vi "Thermocouple DAQ Setup.vi"(0 "task in":refnum<k21>, 1 "sample mode":i32(ring)=10123 items=["Finite Samples"=10178, "Continuous Samples"=10123, "Hardware Timed Single Point"=12522], 3 "Thermocouple Type":i32(ring)=10073 items=["J"=10072, "K"=10073, "N"=10077, "R"=10082, "S"=10085, "T"=10086, "B"=10047, "E"=10055], 5 "physical channels":tag, 7 "Sample Rate":dbl=1000.0 format="%0.2f", 9 "minimum value":dbl format="%0.2f", 11 "error in":errorcluster, 12 "samples per channel":i32=1) -> (4 "task out":refnum<k21>, 15 "error out":errorcluster)   [LabVIEW 2016]
uses:
  <vilib>/DAQmx/create/channels.llb/DAQmx Create Channel (AI-Temperature-Thermocouple).vi
  <vilib>/DAQmx/configure/timing.llb/DAQmx Timing (Sample Clock).vi
panel:
  in  "maximum value":dbl=100.0 format="%0.2f"
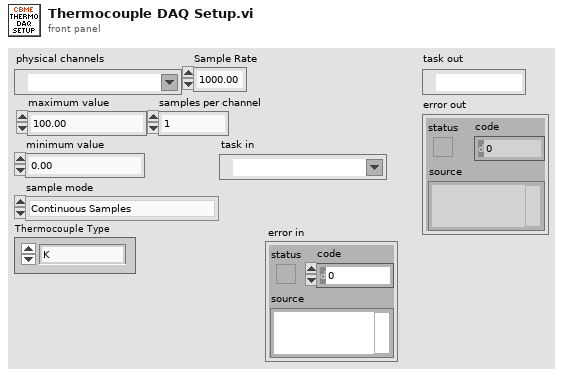
[diagram p1: front panel]
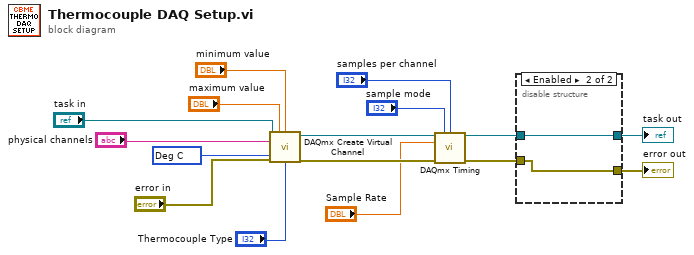
[diagram p0: block diagram]
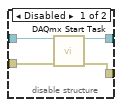
[diagram p2: hidden frame]
diagram:
  w13 = 10143 items=["Deg C"=10143, "Deg F"=10144, "Kelvins"=10325, "Deg R"=10145, "From Custom Scale"=10065] ("units")
  n1 = call-poly <vilib>:"DAQmx Create Virtual Channel.vi"("task in"="task in", "maximum value"="maximum value", "minimum value"="minimum value", "physical channels"="physical channels", "units"=w13, "error in"="error in", "thermocouple type"="Thermocouple Type") -> ("task out"=w12:refnum<k21>, "error out"=w11:errorcluster)  [unwired: 7 in]
  n2 = call-poly <vilib>:"DAQmx Timing.vi"("task/channels in"=w12, "sample mode"="sample mode", "samples per channel"="samples per channel", "rate"="Sample Rate", "error in"=w11) -> ("task out"=w7:refnum<k21>, "error out"=w6:errorcluster)  [unwired: 9 in]
  n3 = disable-structure shown="Enabled" {
    disable-tunnel: w7 -> [w20 w22]
    disable-tunnel: w6 -> [w19 w21]
    disable-tunnel: [w18 w22] -> w5
    disable-tunnel: [w17 w21] -> w4
    frame Disabled {
      n4 = call <vilib>:"DAQmx Start Task.vi"("task/channels in"=w20, "error in"=w19) -> ("task out"=w18:refnum<k21>, "error out"=w17:errorcluster)  [unwired: 12 in]
    }
    frame Enabled {
    }
  }
  "task out" <- w5
  "error out" <- w4
